vi "CloseCom.vi"(8 "error in (no error)":errorcluster, 11 "Data In":T1) -> (0 "error out":errorcluster, 3 "Data Out":T1)   [LabVIEW 2014]
uses:
  controls/Data.ctl
panel:
  # "日期"
  # "機種名稱"
  # "機種代號"
  # "商品條碼"
  # "OK"
  # "台"
  # "NG"
  # "總計"
  # "台"
  # "日期"
  # "機種名稱"
  # "機種代號"
  # "商品條碼"
  # "OK"
  # "台"
  # "NG"
  # "總計"
  # "台"
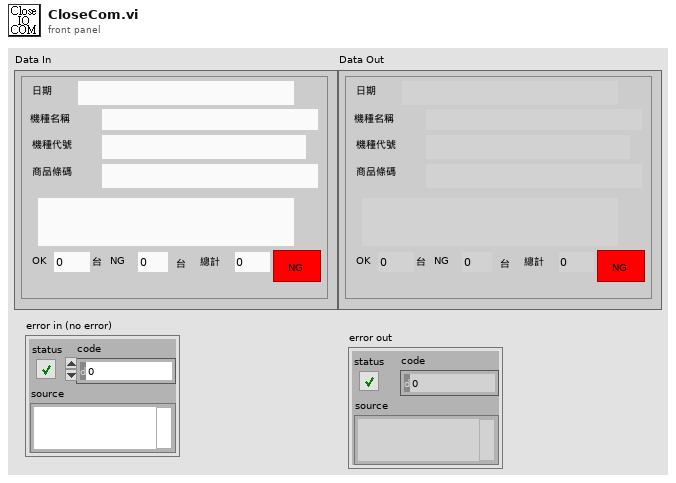
[diagram p1: front panel]
types:
  T1 = typedef "Data.ctl" = cluster{"Date":string, "BarCode1":string, "BarCode2":string, "BarCode3":string, "Message":string, "OK Count":u16, "NG Count":u16, "Total Count":u16, "ModelData":string[][], "OK&NG":bool, "COM1":refnum<visa-resource-name>, "COM2":refnum<visa-resource-name>, "IO":i32, "Time":u32, "TCP":refnum<k5>}
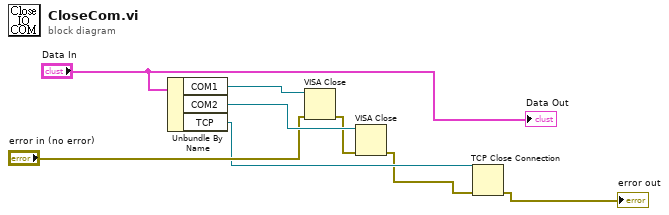
[diagram p0: block diagram]
diagram:
  n1 = Unbundle By Name("Data In") -> ("COM1"=w8:refnum<visa-resource-name>, "COM2"=w7:refnum<visa-resource-name>, "TCP"=w3:refnum<k5>)
  n2 = VISA Close(VISA resource name=w8, error in (no error)="error in (no error)") -> (error out=w6:errorcluster)
  n3 = VISA Close(VISA resource name=w7, error in (no error)=w6) -> (error out=w2:errorcluster)
  n4 = TCP Close Connection(connection ID=w3, error in (no error)=w2) -> (error out=→"error out":errorcluster)  [unwired: 1 in, 1 out]
  "Data Out" <- "Data In"
